vi "Write Buffer.vi"(8 "error in (no error)":errorcluster, 10 "write buffer":string, 11 "UART Actor in":refnum<class "UART Actor.lvclass">) -> (0 "error out":errorcluster, 3 "UART Actor out":refnum<class "UART Actor.lvclass">)   [LabVIEW 2020, in "UART Actor.lvlib" / "UART Actor.lvclass"]
uses:
  UART Actor.lvclass
  C:/Program Files (x86)/National Instruments/LabVIEW 2020/vi.lib/ActorFramework/Actor/Actor.lvclass
  UART Actor Messages/Check Data Buffer Msg/Check Data Buffer Msg.lvclass
  C:/Program Files (x86)/National Instruments/LabVIEW 2020/vi.lib/ActorFramework/Message/Message.lvclass
  <vilib>/ActorFramework/Time-Delayed Send Message/Time-Delay Override Options.ctl
  <vilib>/ActorFramework/Actor/Actor.lvclass/Actor.ctl
  <vilib>/ActorFramework/Message Enqueuer/Message Enqueuer.lvclass/Message Enqueuer.ctl
  UART Actor.lvclass/UART Actor.ctl
  <vilib>/ActorFramework/Message Enqueuer/Init from Existing Queue.vi
  <vilib>/ActorFramework/Message Enqueuer/Message Enqueuer.lvclass
  <vilib>/ActorFramework/Actor/Actor.lvclass
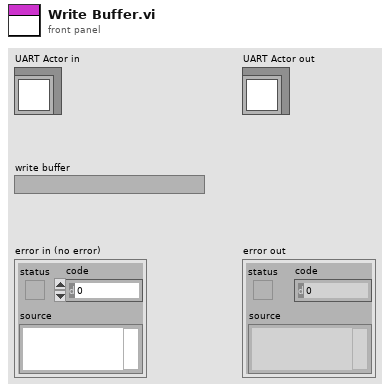
[diagram p1: front panel]
types:
  T1 = typedef "Time-Delay Override Options.ctl" = enum16{"Send next copy now", "Skip next scheduled copy", "Send next copy now and stop all further copies", "Stop all further copies"}
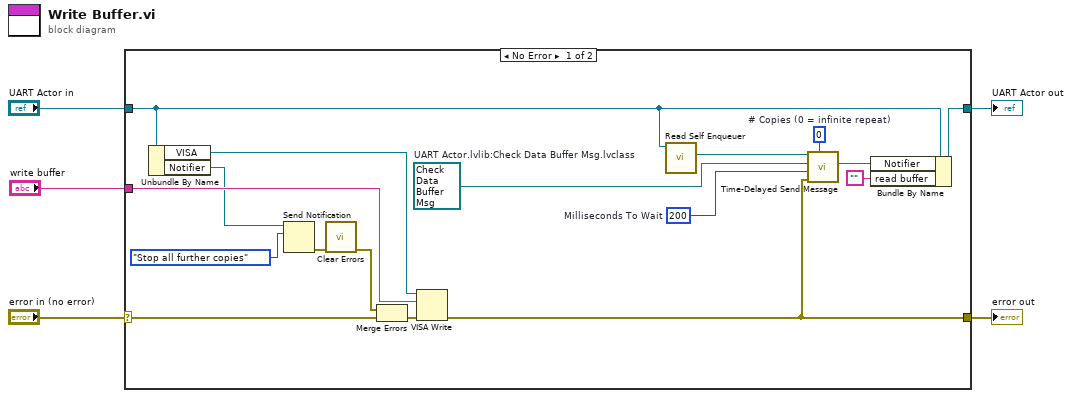
[diagram p0: block diagram]
diagram:
  n1 = case shown="No Error" "error in (no error)" {
    selector: "error in (no error)" -> [w22 w24]
    tunnel: [w9 w24] -> w4
    tunnel: [w19 w23] -> w2
    tunnel: "UART Actor in" -> [w14 w23]
    tunnel: "write buffer" -> [w21 _]
    frame No Error {
      w13 = refnum<class "Check Data Buffer Msg.lvclass"> refnum  # UART Actor.lvlib:Check Data Buffer Msg.lvclass
      w15 = u32 0  # # Copies (0 = infinite repeat)
      w16 = 200  # Milliseconds To Wait
      n2 = Unbundle By Name(w14) -> ("VISA"=w20:refnum<visa-resource-name>, "Notifier"=w12:refnum<notifier>)
      n3 = Send Notification(notification=Time-Delay_Override_Options."Stop all further copies", notifier=w12) -> (error out=w8:errorcluster)  [unwired: 1 in, 1 out]
      n4 = call <vilib>:"Clear Errors.vi"("error in (no error)"=w8) -> ("error out"=w7:errorcluster)  [unwired: 5 in, 1 out]
      n5 = Merge Errors(w7, w22) -> (w10:errorcluster)
      n6 = VISA Write(VISA resource name=w20, write buffer=w21, error in (no error)=w10) -> (error out=w9:errorcluster)  [unwired: 2 out]
      n7 = call <vilib>:"Read Self Enqueuer.vi"("Actor"=w14) -> ("Self Enqueuer"=w17:refnum<class "Message Enqueuer.lvclass">)  [unwired: 10 in]
      n8 = call <vilib>:"Time-Delayed Send Message.vi"("# Copies (0 = infinite repeat)"=w15, "error in (no error)"=w9, "Milliseconds To Wait"=w16, "Message"=w13, "Message Enqueuer"=w17) -> ("Delivery Notifier"=w18:refnum<notifier>)  [unwired: 5 in, 1 out]
      n9 = Bundle By Name(cluster=w14, "Notifier"=w18, "read buffer"="") -> (w19:refnum<class "UART Actor.lvclass">)
    }
    frame Error {
    }
  }
  "error out" <- w4
  "UART Actor out" <- w2
